vi "PicoWriteTDMS.vi"(8 "error in (no error)":errorcluster, 9 "Analog Channels":cluster{i32, sgl, "Data":dbl[]}[](array[cluster])=[{0, 2.4e-08, "Data"=array[5000000 elements]}, {0, 2.4e-08, "Data"=[]}, {0, 2.4e-08, "Data"=[]}, {0, 2.4e-08, "Data"=[]}], 10 "seconds since 1Jan1904":timestamp, 11 "Refnum in":refnum<k34>) -> (0 "error out":errorcluster, 3 "Refnum out":refnum<k34>)   [LabVIEW 2010]
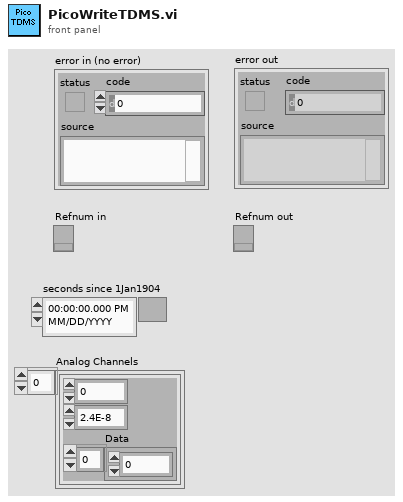
[diagram p1: front panel]
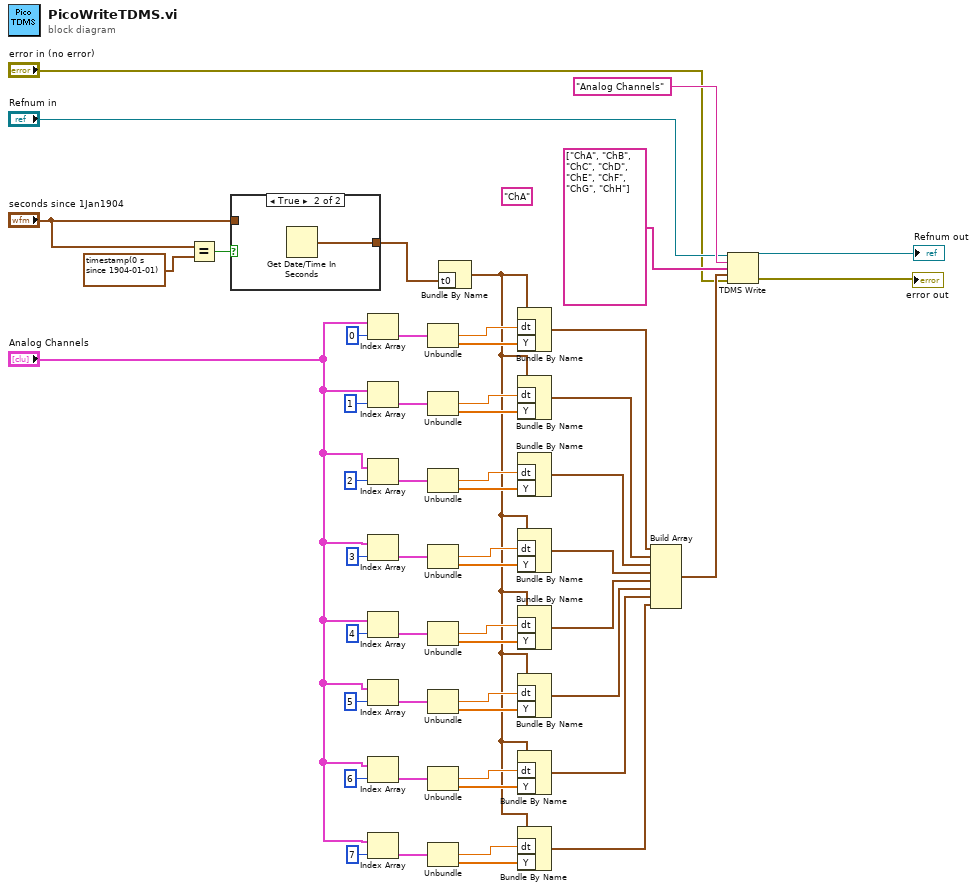
[diagram p0: block diagram]
diagram:
  (unwired) "ChA" ("channel name(s) in (Untitled)")
  n1 = Equal?(x="seconds since 1Jan1904", y=timestamp(0 s since 1904-01-01) ("seconds since 1Jan1904")) -> (x = y?=w3:bool)
  n2 = case shown="True" w3 {
    tunnel: [w54 w55] -> w5
    tunnel: "seconds since 1Jan1904" -> [w54 _]
    frame False {
    }
    frame True {
      n3 = Get Date/Time In Seconds() -> (seconds since 1Jan1904=w55:timestamp)
    }
  }
  n4 = Index Array(array="Analog Channels", index=0) -> (element=w50:cluster{i32, sgl, "Data":dbl[]})
  n5 = Index Array(array="Analog Channels", index=1) -> (element=w47:cluster{i32, sgl, "Data":dbl[]})
  n6 = Index Array(array="Analog Channels", index=2) -> (element=w39:cluster{i32, sgl, "Data":dbl[]})
  n7 = Index Array(array="Analog Channels", index=3) -> (element=w35:cluster{i32, sgl, "Data":dbl[]})
  n8 = Index Array(array="Analog Channels", index=4) -> (element=w31:cluster{i32, sgl, "Data":dbl[]})
  n9 = Index Array(array="Analog Channels", index=5) -> (element=w28:cluster{i32, sgl, "Data":dbl[]})
  n10 = Index Array(array="Analog Channels", index=6) -> (element=w24:cluster{i32, sgl, "Data":dbl[]})
  n11 = Index Array(array="Analog Channels", index=7) -> (element=w20:cluster{i32, sgl, "Data":dbl[]})
  n12 = Unbundle(w50) -> (w49:sgl, "Data"=w48:dbl[])  [unwired: 1 out]
  n13 = Unbundle(w47) -> (w46:sgl, "Data"=w45:dbl[])  [unwired: 1 out]
  n14 = Unbundle(w39) -> (w38:sgl, "Data"=w37:dbl[])  [unwired: 1 out]
  n15 = Unbundle(w35) -> (w34:sgl, "Data"=w33:dbl[])  [unwired: 1 out]
  n16 = Unbundle(w31) -> (w30:sgl, "Data"=w29:dbl[])  [unwired: 1 out]
  n17 = Unbundle(w28) -> (w27:sgl, "Data"=w26:dbl[])  [unwired: 1 out]
  n18 = Unbundle(w24) -> (w23:sgl, "Data"=w22:dbl[])  [unwired: 1 out]
  n19 = Unbundle(w20) -> (w19:sgl, "Data"=w18:dbl[])  [unwired: 1 out]
  n20 = Bundle By Name("t0"=w5) -> (w8:waveform(dbl))  [unwired: 1 in]
  n21 = Bundle By Name(cluster=w8, "dt"=w49, "Y"=w48) -> (w43:waveform(dbl))
  n22 = Bundle By Name(cluster=w8, "dt"=w46, "Y"=w45) -> (w42:waveform(dbl))
  n23 = Bundle By Name("dt"=w38, "Y"=w37) -> (w11:waveform(dbl))  [unwired: 1 in]
  n24 = Bundle By Name(cluster=w8, "dt"=w34, "Y"=w33) -> (w12:waveform(dbl))
  n25 = Bundle By Name(cluster=w8, "dt"=w30, "Y"=w29) -> (w13:waveform(dbl))
  n26 = Bundle By Name(cluster=w8, "dt"=w27, "Y"=w26) -> (w14:waveform(dbl))
  n27 = Bundle By Name(cluster=w8, "dt"=w23, "Y"=w22) -> (w15:waveform(dbl))
  n28 = Bundle By Name(cluster=w8, "dt"=w19, "Y"=w18) -> (w16:waveform(dbl))
  n29 = Build Array(w43, w42, w11, w12, w13, w14, w15, w16) -> (w41:waveform(dbl)[])
  n30 = TDMS Write(0:"Refnum in", 5:"Analog Channels" ("group name in (Untitled)"), 7:string[] ["ChA", "ChB", "ChC", "ChD", "ChE", "ChF", "ChG", "ChH"] ("channel names"), 9:w41, 11:"error in (no error)") -> (4:→"Refnum out":refnum<k34>, 15:→"error out":errorcluster)  [unwired: 1 in, 2 out]
